vi "Instrument Do Core.vi"(8 "error in (no error)":errorcluster, 9 "Instrument in":refnum<class "Instrument Driver.lvclass">, 10 "Actor in":refnum<class "Actor.lvclass">, 11 "Instrument Msg in":refnum<class "Calibrate Instrument Msg.lvclass">) -> (0 "error out":errorcluster, 1 "Instrument out":refnum<class "Instrument Driver.lvclass">, 2 "Actor out":refnum<class "Actor.lvclass">, 3 "Instrument Msg out":refnum<class "Calibrate Instrument Msg.lvclass">, 5 "Data":refnum<class "Data.lvclass">)   [LabVIEW 2020, in "Instrument Handler.lvlib" / "Calibrate Instrument Msg.lvclass"]
doc: "Message interaction with any instrument is handled by the Instrument Do Core.\n\nThis implementation runs the Calibrate method on the Instrument."
uses:
  Calibrate Instrument Msg.lvclass
  PPL/HDH.Actor Framework.Core.Actor.lvlibp/1abvi3w/vi.lib/ActorFramework/Actor/Actor.lvclass
  PPL/HDH.Data.Generic.lvlibp/Data.lvclass
  PPL/HDH.Actor Framework.Core.Instrument Driver.lvlibp/Instrument Driver/Instrument Driver.lvclass
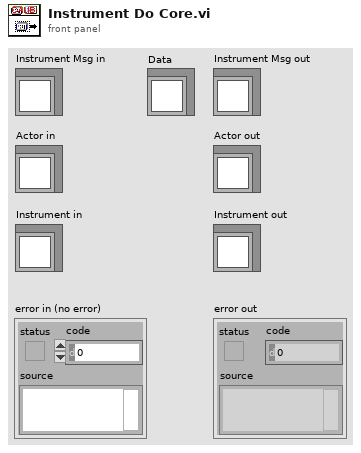
[diagram p1: front panel]
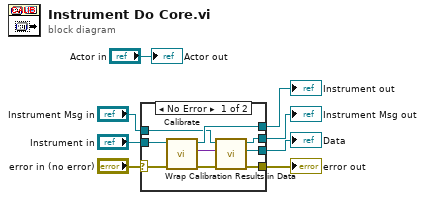
[diagram p0: block diagram]
diagram:
  n1 = case shown="No Error" "error in (no error)" {
    selector: "error in (no error)" -> [w15 w18]
    tunnel: "Instrument in" -> [w17 w20]
    tunnel: [w16 w20] -> w6
    tunnel: [w13 w18] -> w4
    tunnel: "Instrument Msg in" -> [w11 w19]
    tunnel: [w10 w19] -> w2
    tunnel: [w9 _] -> w1
    frame No Error {
      n2 = call-dynamic "Calibrate.vi"("error in (no error)"=w15, "Instrument in"=w17) -> ("error out"=w14:errorcluster, "Result"=w12:variant, "Instrument out"=w16:refnum<class "Instrument Driver.lvclass">)  [unwired: 6 in, 1 out]
      n3 = call-dynamic "Wrap Calibration Results in Data.vi"("error in (no error)"=w14, "Calibration Result"=w12, "Calibrate Instrument Msg in"=w11) -> ("error out"=w13:errorcluster, "Data"=w9:refnum<class "Data.lvclass">, "Calibrate Instrument Msg out"=w10:refnum<class "Calibrate Instrument Msg.lvclass">)  [unwired: 6 in]
    }
    frame Error {
    }
  }
  "error out" <- w4
  "Instrument Msg out" <- w2
  "Instrument out" <- w6
  "Data" <- w1
  "Actor out" <- "Actor in"
